vi "FPGA_UtilitiesWrite LED.vi"(8 "error in (no error)":errorcluster, 11 "FPGA LED":bool) -> (0 "error out":errorcluster)   [LabVIEW 2017]
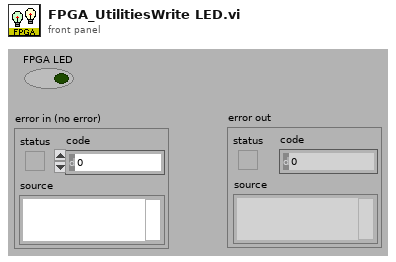
[diagram p1: front panel]
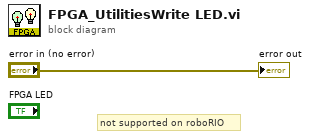
[diagram p0: block diagram]
diagram:
  # "not supported on roboRIO"
  "error out" <- "error in (no error)"
